vi "Read Shared Variable - General - Refnum.vi"(8 "Error In":errorcluster, 9 "Type code":i32, 10 "Refnum":refnum<k21>) -> (0 "Error Out":errorcluster, 1 "Data":variant, 2 "size(s)":i32[](array[numeric]), 3 "Size":string)   [LabVIEW 2014]
doc: "<B>Copyright</B>: (c) MHWirth 2015. All rights are reserved.\n\nThis SubVI reads the shared variable and returns it as a variant. It returns the size of the variable in two formats: numeric and string.\n\n<B>Note 2</B>: It does not support 1D and 2D arrays of <B>strings</B>.\n\n\nSupported shared variable types:\nCode 1. Boolean\nCode 2 to 5. Int8/16/32/64\nCode 6 to 9. UInt8/16/32/64\nCode 10. Double\nCode 11. Single-precision\nCode 12. String\nCode 13-23 - 1D array of above types except string\n\n<B>Error 7001</B>: Unknown Data Type - Type Code Array (Int32) contains -1 indicating an unknown data type."
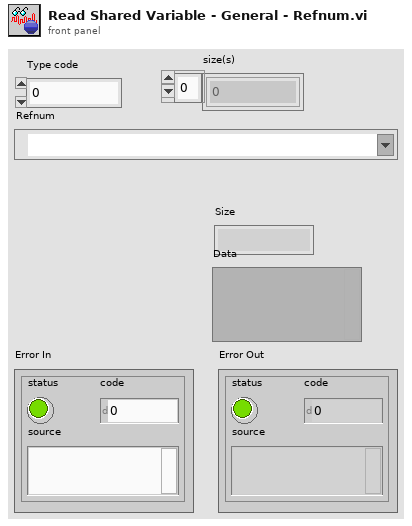
[diagram p1: front panel]
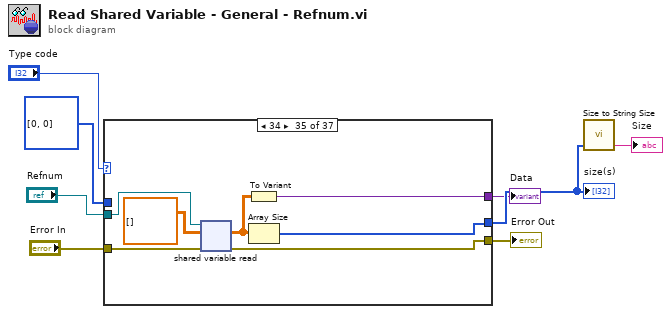
[diagram p0: block diagram]
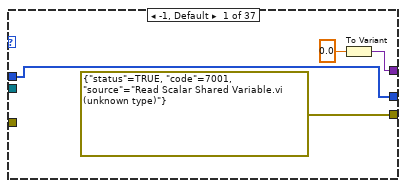
[diagram p2: hidden frame]
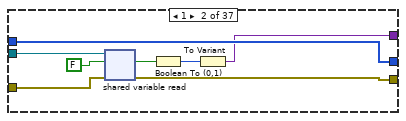
[diagram p3: hidden frame]
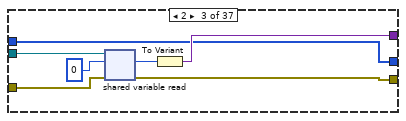
[diagram p4: hidden frame]
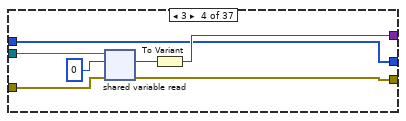
[diagram p5: hidden frame]
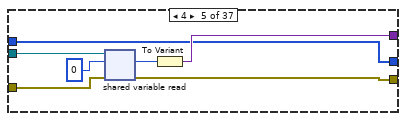
[diagram p6: hidden frame]
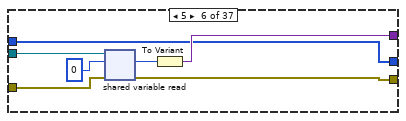
[diagram p7: hidden frame]
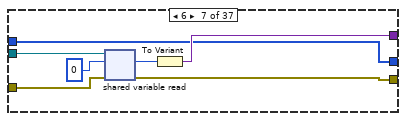
[diagram p8: hidden frame]
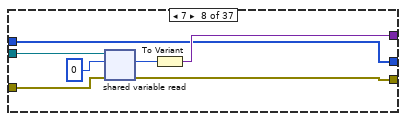
[diagram p9: hidden frame]
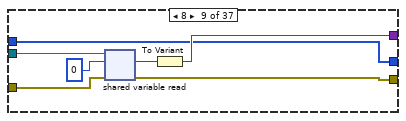
[diagram p10: hidden frame]
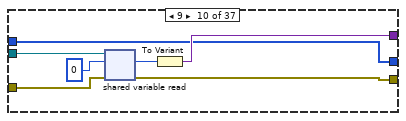
[diagram p11: hidden frame]
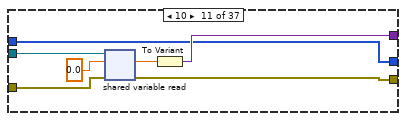
[diagram p12: hidden frame]
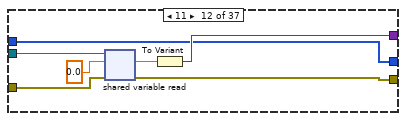
[diagram p13: hidden frame]
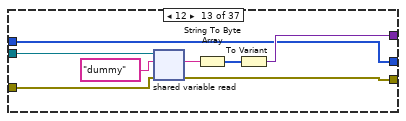
[diagram p14: hidden frame]
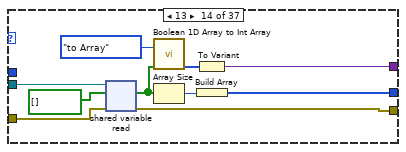
[diagram p15: hidden frame]
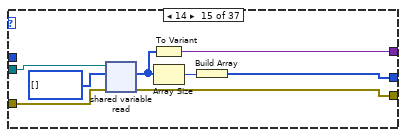
[diagram p16: hidden frame]
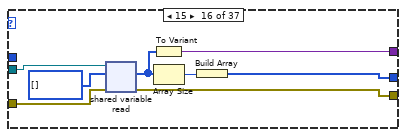
[diagram p17: hidden frame]
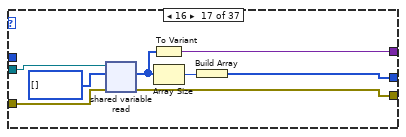
[diagram p18: hidden frame]
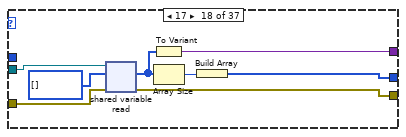
[diagram p19: hidden frame]
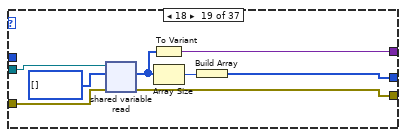
[diagram p20: hidden frame]
diagram:
  n1 = case shown="34" "Type code" {
    tunnel: [errorcluster {"status"=TRUE, "code"=7001, "source"="Read Scalar Shared Variable.vi (unknown type)"} ("error constant") w19 w26 w33 w40 w47 w54 w61 w68 w75 w82 w89 w98 w108 w116 w124 w132 w140 w148 w156 w164 w172 w180 w188 errorcluster {"status"=FALSE, "code"=7002, "source"="Read Shared Variable.vi (1D array of string not supported)"} ("Error In") w201 w208 w215 w222 w229 w236 w243 w250 w257 w264 w271 errorcluster {"status"=FALSE, "code"=7003, "source"="Read Shared Variable.vi (2D array of string not supported)"} ("Error In")] -> w7
    tunnel: "Refnum" -> [_ w18 w24 w31 w38 w45 w52 w59 w66 w73 w80 w87 w96 w106 w114 w122 w130 w138 w146 w154 w162 w170 w178 w186 _ w199 w206 w213 w220 w227 w234 w241 w248 w255 w262 w269 _]
    tunnel: "Error In" -> [_ w17 w25 w32 w39 w46 w53 w60 w67 w74 w81 w88 w97 w107 w115 w123 w131 w139 w147 w155 w163 w171 w179 w187 _ w200 w207 w214 w221 w228 w235 w242 w249 w256 w263 w270 _]
    tunnel: [w11 w15 w21 w28 w35 w42 w49 w56 w63 w70 w77 w84 w91 w99 w109 w119 w127 w135 w141 w149 w157 w165 w174 w181 w189 w193 w202 w209 w216 w223 w231 w237 w245 w252 w259 w265 w272] -> w3
    tunnel: i32[] [0, 0] ("size(s)") -> [w11 w15 w21 w28 w35 w42 w49 w56 w63 w70 w77 w84 w91 _ _ _ _ _ _ _ _ _ _ _ w189 _ _ _ _ _ _ _ _ _ _ _ w272]
    tunnel: [w9 w13 w22 w30 w36 w43 w50 w57 w64 w71 w78 w85 w92 w102 w112 w120 w128 w136 w144 w152 w160 w168 w176 w184 w191 w195 w204 w211 w218 w225 w232 w239 w246 w253 w260 w267 w273] -> w1
    frame -1, Default {
      n2 = To Variant(anything=0.0) -> (Variant=w9:variant)
    }
    frame 1 {
      n3 = shared-variable-read(w18, w17, FALSE) -> (w19:errorcluster, w16:bool)  [unwired: 2 out]
      n4 = Boolean To (0,1)(Boolean=w16) -> (0, 1=w14:i16)
      n5 = To Variant(anything=w14) -> (Variant=w13:variant)
    }
    frame 2 {
      n6 = shared-variable-read(w24, w25, i8 0) -> (w26:errorcluster, w23:i8)  [unwired: 2 out]
      n7 = To Variant(anything=w23) -> (Variant=w22:variant)
    }
    frame 3 {
      n8 = shared-variable-read(w31, w32, i16 0) -> (w33:errorcluster, w29:i16)  [unwired: 2 out]
      n9 = To Variant(anything=w29) -> (Variant=w30:variant)
    }
    frame 4 {
      n10 = shared-variable-read(w38, w39, 0) -> (w40:errorcluster, w37:i32)  [unwired: 2 out]
      n11 = To Variant(anything=w37) -> (Variant=w36:variant)
    }
    frame 5 {
      n12 = shared-variable-read(w45, w46, i64 0) -> (w47:errorcluster, w44:i64)  [unwired: 2 out]
      n13 = To Variant(anything=w44) -> (Variant=w43:variant)
    }
    frame 6 {
      n14 = shared-variable-read(w52, w53, u8 0) -> (w54:errorcluster, w51:u8)  [unwired: 2 out]
      n15 = To Variant(anything=w51) -> (Variant=w50:variant)
    }
    frame 7 {
      n16 = shared-variable-read(w59, w60, u16 0) -> (w61:errorcluster, w58:u16)  [unwired: 2 out]
      n17 = To Variant(anything=w58) -> (Variant=w57:variant)
    }
    frame 8 {
      n18 = shared-variable-read(w66, w67, u32 0) -> (w68:errorcluster, w65:u32)  [unwired: 2 out]
      n19 = To Variant(anything=w65) -> (Variant=w64:variant)
    }
    frame 9 {
      n20 = shared-variable-read(w73, w74, u64 0) -> (w75:errorcluster, w72:u64)  [unwired: 2 out]
      n21 = To Variant(anything=w72) -> (Variant=w71:variant)
    }
    frame 10 {
      n22 = shared-variable-read(w80, w81, 0.0) -> (w82:errorcluster, w79:dbl)  [unwired: 2 out]
      n23 = To Variant(anything=w79) -> (Variant=w78:variant)
    }
    frame 11 {
      n24 = shared-variable-read(w87, w88, sgl 0.0) -> (w89:errorcluster, w86:sgl)  [unwired: 2 out]
      n25 = To Variant(anything=w86) -> (Variant=w85:variant)
    }
    frame 12 {
      n26 = shared-variable-read(w96, w97, "dummy") -> (w98:errorcluster, w94:string)  [unwired: 2 out]
      n27 = String To Byte Array(string=w94) -> (unsigned byte array=w93:u8[])
      n28 = To Variant(anything=w93) -> (Variant=w92:variant)
    }
    frame 13 {
      n29 = shared-variable-read(w106, w107, bool[] []) -> (w108:errorcluster, w101:bool[])  [unwired: 2 out]
      n30 = call "Boolean 1D Array to Int Array.vi"("Mode"=enum16{"to Array", "to Number"}."to Array" ("Enum"), "Array of Boolean"=w101) -> ("Array out"=w103:u32[])  [unwired: 8 in]
      n31 = Array Size(array=w101) -> (size(s)=w100:i32)
      n32 = To Variant(anything=w103) -> (Variant=w102:variant)
      n33 = Build Array(w100) -> (w99:i32[])
    }
    frame 14 {
      n34 = shared-variable-read(w114, w115, i8[] []) -> (w116:errorcluster, w111:i8[])  [unwired: 2 out]
      n35 = To Variant(anything=w111) -> (Variant=w112:variant)
      n36 = Array Size(array=w111) -> (size(s)=w110:i32)
      n37 = Build Array(w110) -> (w109:i32[])
    }
    frame 15 {
      n38 = shared-variable-read(w122, w123, i16[] []) -> (w124:errorcluster, w117:i16[])  [unwired: 2 out]
      n39 = To Variant(anything=w117) -> (Variant=w120:variant)
      n40 = Array Size(array=w117) -> (size(s)=w118:i32)
      n41 = Build Array(w118) -> (w119:i32[])
    }
    frame 16 {
      n42 = shared-variable-read(w130, w131, i32[] []) -> (w132:errorcluster, w125:i32[])  [unwired: 2 out]
      n43 = To Variant(anything=w125) -> (Variant=w128:variant)
      n44 = Array Size(array=w125) -> (size(s)=w126:i32)
      n45 = Build Array(w126) -> (w127:i32[])
    }
    frame 17 {
      n46 = shared-variable-read(w138, w139, i64[] []) -> (w140:errorcluster, w133:i64[])  [unwired: 2 out]
      n47 = To Variant(anything=w133) -> (Variant=w136:variant)
      n48 = Array Size(array=w133) -> (size(s)=w134:i32)
      n49 = Build Array(w134) -> (w135:i32[])
    }
    frame 18 {
      n50 = shared-variable-read(w146, w147, u8[] []) -> (w148:errorcluster, w143:u8[])  [unwired: 2 out]
      n51 = To Variant(anything=w143) -> (Variant=w144:variant)
      n52 = Array Size(array=w143) -> (size(s)=w142:i32)
      n53 = Build Array(w142) -> (w141:i32[])
    }
    frame 19 {
      n54 = shared-variable-read(w154, w155, u16[] []) -> (w156:errorcluster, w151:u16[])  [unwired: 2 out]
      n55 = To Variant(anything=w151) -> (Variant=w152:variant)
      n56 = Array Size(array=w151) -> (size(s)=w150:i32)
      n57 = Build Array(w150) -> (w149:i32[])
    }
    frame 20 {
      n58 = shared-variable-read(w162, w163, u32[] []) -> (w164:errorcluster, w159:u32[])  [unwired: 2 out]
      n59 = To Variant(anything=w159) -> (Variant=w160:variant)
      n60 = Array Size(array=w159) -> (size(s)=w158:i32)
      n61 = Build Array(w158) -> (w157:i32[])
    }
    frame 21 {
      n62 = shared-variable-read(w170, w171, u64[] []) -> (w172:errorcluster, w167:u64[])  [unwired: 2 out]
      n63 = To Variant(anything=w167) -> (Variant=w168:variant)
      n64 = Array Size(array=w167) -> (size(s)=w166:i32)
      n65 = Build Array(w166) -> (w165:i32[])
    }
    frame 22 {
      n66 = shared-variable-read(w178, w179, dbl[] []) -> (w180:errorcluster, w173:dbl[])  [unwired: 2 out]
      n67 = To Variant(anything=w173) -> (Variant=w176:variant)
      n68 = Array Size(array=w173) -> (size(s)=w175:i32)
      n69 = Build Array(w175) -> (w174:i32[])
    }
    frame 23 {
      n70 = shared-variable-read(w186, w187, sgl[] []) -> (w188:errorcluster, w183:sgl[])  [unwired: 2 out]
      n71 = To Variant(anything=w183) -> (Variant=w184:variant)
      n72 = Array Size(array=w183) -> (size(s)=w182:i32)
      n73 = Build Array(w182) -> (w181:i32[])
    }
    frame 24 {
      n74 = To Variant(anything=0.0) -> (Variant=w191:variant)
    }
    frame 25 {
      n75 = shared-variable-read(w199, w200, bool[][] []) -> (w201:errorcluster, w194:bool[][])  [unwired: 2 out]
      n76 = call "Boolean 2D Array to Int Array.vi"("Mode"=enum16{"to Array", "to Number"}."to Array" ("Enum"), "Array of Boolean"=w194) -> ("Array out"=w196:u32[][])  [unwired: 8 in]
      n77 = Array Size(array=w194) -> (size(s)=w193:i32[])
      n78 = To Variant(anything=w196) -> (Variant=w195:variant)
    }
    frame 26 {
      n79 = shared-variable-read(w206, w207, i8[][] []) -> (w208:errorcluster, w203:i8[][])  [unwired: 2 out]
      n80 = To Variant(anything=w203) -> (Variant=w204:variant)
      n81 = Array Size(array=w203) -> (size(s)=w202:i32[])
    }
    frame 27 {
      n82 = shared-variable-read(w213, w214, i16[][] []) -> (w215:errorcluster, w210:i16[][])  [unwired: 2 out]
      n83 = To Variant(anything=w210) -> (Variant=w211:variant)
      n84 = Array Size(array=w210) -> (size(s)=w209:i32[])
    }
    frame 28 {
      n85 = shared-variable-read(w220, w221, i32[][] []) -> (w222:errorcluster, w217:i32[][])  [unwired: 2 out]
      n86 = To Variant(anything=w217) -> (Variant=w218:variant)
      n87 = Array Size(array=w217) -> (size(s)=w216:i32[])
    }
    frame 29 {
      n88 = shared-variable-read(w227, w228, i64[][] []) -> (w229:errorcluster, w224:i64[][])  [unwired: 2 out]
      n89 = To Variant(anything=w224) -> (Variant=w225:variant)
      n90 = Array Size(array=w224) -> (size(s)=w223:i32[])
    }
    frame 30 {
      n91 = shared-variable-read(w234, w235, u8[][] []) -> (w236:errorcluster, w230:u8[][])  [unwired: 2 out]
      n92 = To Variant(anything=w230) -> (Variant=w232:variant)
      n93 = Array Size(array=w230) -> (size(s)=w231:i32[])
    }
    frame 31 {
      n94 = shared-variable-read(w241, w242, u16[][] []) -> (w243:errorcluster, w238:u16[][])  [unwired: 2 out]
      n95 = To Variant(anything=w238) -> (Variant=w239:variant)
      n96 = Array Size(array=w238) -> (size(s)=w237:i32[])
    }
    frame 32 {
      n97 = shared-variable-read(w248, w249, u32[][] []) -> (w250:errorcluster, w244:u32[][])  [unwired: 2 out]
      n98 = To Variant(anything=w244) -> (Variant=w246:variant)
      n99 = Array Size(array=w244) -> (size(s)=w245:i32[])
    }
    frame 33 {
      n100 = shared-variable-read(w255, w256, u64[][] []) -> (w257:errorcluster, w251:u64[][])  [unwired: 2 out]
      n101 = To Variant(anything=w251) -> (Variant=w253:variant)
      n102 = Array Size(array=w251) -> (size(s)=w252:i32[])
    }
    frame 34 {
      n103 = shared-variable-read(w262, w263, dbl[][] []) -> (w264:errorcluster, w258:dbl[][])  [unwired: 2 out]
      n104 = To Variant(anything=w258) -> (Variant=w260:variant)
      n105 = Array Size(array=w258) -> (size(s)=w259:i32[])
    }
    frame 35 {
      n106 = shared-variable-read(w269, w270, sgl[][] []) -> (w271:errorcluster, w266:sgl[][])  [unwired: 2 out]
      n107 = To Variant(anything=w266) -> (Variant=w267:variant)
      n108 = Array Size(array=w266) -> (size(s)=w265:i32[])
    }
    frame 36 {
      n109 = To Variant(anything=0.0) -> (Variant=w273:variant)
    }
  }
  "Error Out" <- w7
  "size(s)" <- w3
  "Data" <- w1
  n110 = call "Size to String Size.vi"("size(s)"=w3) -> ("Size"=→"Size":string)  [unwired: 4 in]
